vi "Calibration Output.vi"(1 "Input":dbl, 2 "Calibration Output FGV Selector":T1, 3 "Action":T2) -> (0 "Output":dbl)   [LabVIEW 2013]
uses:
  Action.ctl
  Calibration Output FGV Selector.ctl
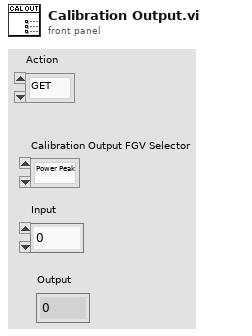
[diagram p1: front panel]
types:
  T1 = typedef "Calibration Output FGV Selector.ctl" = enum16{"Power Peak", "Slope", "Spring Constant"}
  T2 = typedef "Action.ctl" = enum16{"GET", "PUT", "DELETE"}
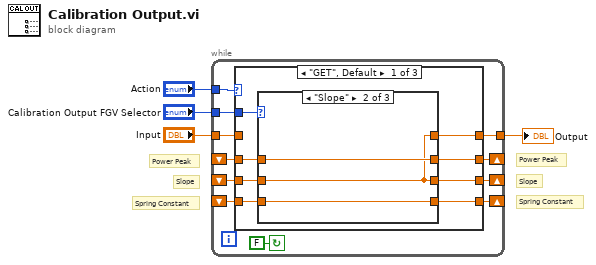
[diagram p0: block diagram]
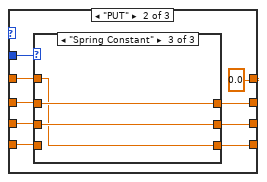
[diagram p4: hidden frame]
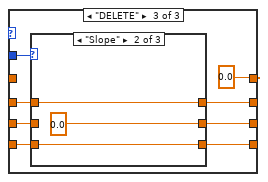
[diagram p7: hidden frame]
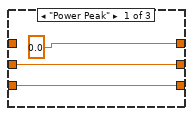
[diagram p8: hidden frame]
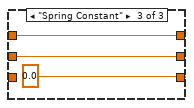
[diagram p9: hidden frame]
diagram:
  # "Spring Constant"
  # "Slope"
  # "Power Peak"
  # "Spring Constant"
  # "Slope"
  # "Power Peak"
  n1 = while {
    tunnel: "Action" -> [w14]
    tunnel: "Input" -> [w13]
    tunnel: [w12] -> w2
    shift-right: [w10] -> _
    shift-left: _ -> [w9]
    shift-right: [w8] -> _
    shift-left: _ -> [w7]
    shift-right: [w5] -> _
    shift-left: _ -> [w6]
    tunnel: "Calibration Output FGV Selector" -> [w11]
    stop <- FALSE continue-if-true
    n2 = case shown="\"GET\", Default" w14 {
      tunnel: w13 -> [_ w34 _]
      tunnel: [w16 0.0 0.0] -> w12
      tunnel: w11 -> [w23 w33 w51]
      tunnel: [w22 w37 w54] -> w10
      tunnel: w9 -> [w21 w41 w57]
      tunnel: [w20 w36 w53] -> w8
      tunnel: w7 -> [w19 w40 w56]
      tunnel: w6 -> [w17 w39 w55]
      tunnel: [w18 w35 w52] -> w5
      frame "GET", Default {
        n3 = case shown="\"Slope\"" w23 {
          tunnel: [w24 w29 w32] -> w22
          tunnel: w21 -> [w24 w29 w32]
          tunnel: [w26 w27 w31] -> w20
          tunnel: w19 -> [w26 w27 w31]
          tunnel: [w25 w28 w30] -> w18
          tunnel: w17 -> [w25 w28 w30]
          tunnel: [w24 w27 w30] -> w16
          frame "Power Peak" {
          }
          frame "Slope" {
          }
          frame "Spring Constant" {
          }
        }
      }
      frame "PUT" {
        n4 = case shown="\"Spring Constant\"" w33 {
          tunnel: [w42 w47 w50] -> w37
          tunnel: w41 -> [_ w47 w50]
          tunnel: [w44 w45 w49] -> w36
          tunnel: w40 -> [w44 _ w49]
          tunnel: [w43 w46 w48] -> w35
          tunnel: w39 -> [w43 w46 _]
          tunnel: w34 -> [w42 w45 w48]
          frame "Power Peak" {
          }
          frame "Slope" {
          }
          frame "Spring Constant" {
          }
        }
      }
      frame "DELETE" {
        n5 = case shown="\"Slope\"" w51 {
          tunnel: [0.0 w64 w67] -> w54
          tunnel: w57 -> [_ w64 w67]
          tunnel: [w61 0.0 w66] -> w53
          tunnel: w56 -> [w61 _ w66]
          tunnel: [w60 w63 0.0] -> w52
          tunnel: w55 -> [w60 w63 _]
          frame "Power Peak" {
          }
          frame "Slope" {
          }
          frame "Spring Constant" {
          }
        }
      }
    }
  }
  "Output" <- w2
